vi "Old OM Setup.vi"() -> ()   [LabVIEW 2013]
uses:
  lib/Data Access Objects/Metadata/Persistant DAO Actions.ctl
  lib/Data Access Objects/Metadata/LBCB Number.ctl
  Popups/External Sensor Specs.ctl
  lib/Data Access Objects/Application/Number Of LBCBs.ctl
  Popups/Update Table Actions.ctl
  lib/Data Access Objects/Metadata/LBCB Location.ctl
  lib/Data Access Objects/Metadata/Actuator Point.ctl
  lib/Data Access Objects/Metadata/Actuator Matrix.ctl
  lib/Data Access Objects/Metadata/Cartesian Point.ctl
  lib/Data Access Objects/Metadata/Cartesian Matrix.ctl
  lib/Data Access Objects/Application/Timing Parameters.ctl
  lib/Data Access Objects/Application/App Parameters.ctl
  lib/Data Access Objects/Metadata/LBCB Position.ctl
  lib/MixedMode/Stiffness Matrix.ctl
  lib/Data Access Objects/Limits/Limit Boundary Parameters.ctl
  lib/Data Access Objects/Autobalance/Autobalance Control Parameters.ctl
  lib/Data Access Objects/Metadata/Actuator Channel Names.ctl
  lib/MixedMode/Ramp Control.ctl
  lib/MixedMode/Ramp Time Input.ctl
  lib/Data Access Objects/Metadata/Cartesian Force Vector.ctl
  lib/Data Access Objects/Application/Network Parameters.ctl
  lib/Data Access Objects/Mixed Mode/Force Control Parameters.ctl
  lib/Data Access Objects/Metadata/Cartesian Force Matrix.ctl
  lib/Data Access Objects/Metadata/Pin Positions.ctl
panel:
  out "Profile":string
  in  "Rigid Connection":bool
  in  "LBCB Number Button":bool
  in  "Number of LBCBs":T1
  in  "Save":bool
  in  "OM Setup Page Tab":T2(tab)
  in  "Act Incr Limit":T3 caption="Increment Limits"
  in  "Act Disp Bnd":T4 caption="Actuator Disp Limit \nBoundary Parameters"
  in  "Actuator Force Limits":T5
  in  "Actuator Stroke Limits":T5
  in  "Command Voltage Limit":T5
  in  "Act Force Bnd":T4 caption="Actuator Force Limit \nBoundary Parameters"
  in  "Cart Incr Limits":T6 caption="Increment Limits"
  in  "Cartesian Displacement Limits":T7
  in  "Cartesian Force Limits":T7
  in  "Cart Force Bnd":T4 caption="Cartesian Force Limit \nBoundary Parameters"
  in  "Cart Trans Bnd":T4 caption="Cartesian Translation Limit \nBoundary Parameters"
  in  "Cart Rot Bnd":T4 caption="Cartesian Rotation Limit \nBoundary Parameters"
  in  "Cart Mmt Bnd":T4 caption="Cartesian Moment Limit \nBoundary Parameters"
  in  "Auto Balance Control":T8={"Number of Samples"=0, "Delay After Cmd"=0, "Maximum Command"=0.0, "1/4 Linear Range"=0.5}
  in  "Auto Balance Error Window":T3
  in  "I Gain":T3
  in  "P Gain":T3
  in  "NTCP Network":T9={"Port Number"=0, "Notification Name"="DataAvailableForTransmission", "Wait For Notification Timeout"=1000}
  in  "DAQ Link Network":T9={"Port Number"=0, "Notification Name"="DataAvailableForTransmission", "Wait For Notification Timeout"=1000}
  in  "Application Timing and Logging":T10
  in  "Ramp Times":T12
  in  "LBCB Pin Positions":T14
  in  "LBCB Position":T15={"Motion Center"=[0.0, 0.0, 0.0], "Transformation Matrix"=[[1.0, 0.0, 0.0, 0.0, 0.0, 0.0], [0.0, 1.0, 0.0, 0.0, 0.0, 0.0], [0.0, 0.0, 1.0, 0.0, 0.0, 0.0], [0.0, 0.0, 0.0, 1.0, 0.0, 0.0], [0.0, 0.0, 0.0, 0.0, 1.0, 0.0], [0.0, 0.0, 0.0, 0.0, 0.0, 1.0]]} {"Transformation Matrix" format="%#_10e"; "Motion Center" format="%#_10g"}
  in  "Force Control Parameters":T16
  in  "Stiffness Limit":T17
  in  "Force Group Priorities":T18
  in  "Force Error Range":T18
  in  "Jacobian Gain":T6
  in  "Max Increment":T6
  in  "Stiffness Jacobian":T19=[[1000000.0, 0.0, 0.0, 0.0, 0.0, 0.0], [0.0, 1000000.0, 0.0, 0.0, 0.0, 0.0], [0.0, 0.0, 1000000.0, 0.0, 0.0, 0.0], [0.0, 0.0, 0.0, 1000000.0, 0.0, 0.0], [0.0, 0.0, 0.0, 0.0, 1000000.0, 0.0], [0.0, 0.0, 0.0, 0.0, 0.0, 1000000.0]]
  in  "Servo Error Offset":T3
  in  "LVDT  Offset":T3
  in  "Load Cell  Offset":T3
  in  "Load Cell Sensitivity":T3
  in  "Command Sensitivity":T3
  in  "LVDT Sensitivity":T3
  in  "Command Channels":T20
  in  "LVDT Channels":T20
  in  "Load Cell Channels":T20
  in  "Servo Error  Channels":T20
  in  "External Sensor Specs":T21[](array[typedef])
  out "OM  Location":T22
  in  "Ok":bool
  in  "LBCB Number":T23
  # "(Volts)"
  # "Interval is in Seconds\nRate is in Samples per Second"
  # "Fixed"
  # "Platten"
  # "X"
  # "Z"
  # "X"
  # "Z"
  # "Y"
  # "Y"
  # "Y"
  # "(inch)"
  # "XLBCB CMD = T-1*XLBCB OM"
  # "Z"
  # "(inch)"
  # "XOM DISP = T*XLBCB DISP"
  # "(inch)"
  # "Dx"
  # "Dy"
  # "Dz"
  # "Rx"
  # "Ry"
  # "Rz"
  # "Dx"
  # "Dy"
  # "Dz"
  # "Rx"
  # "Ry"
  # "Rz"
  # "DAQMx Global Channel"
  # "Display Name"
  # "Sensiitivity"
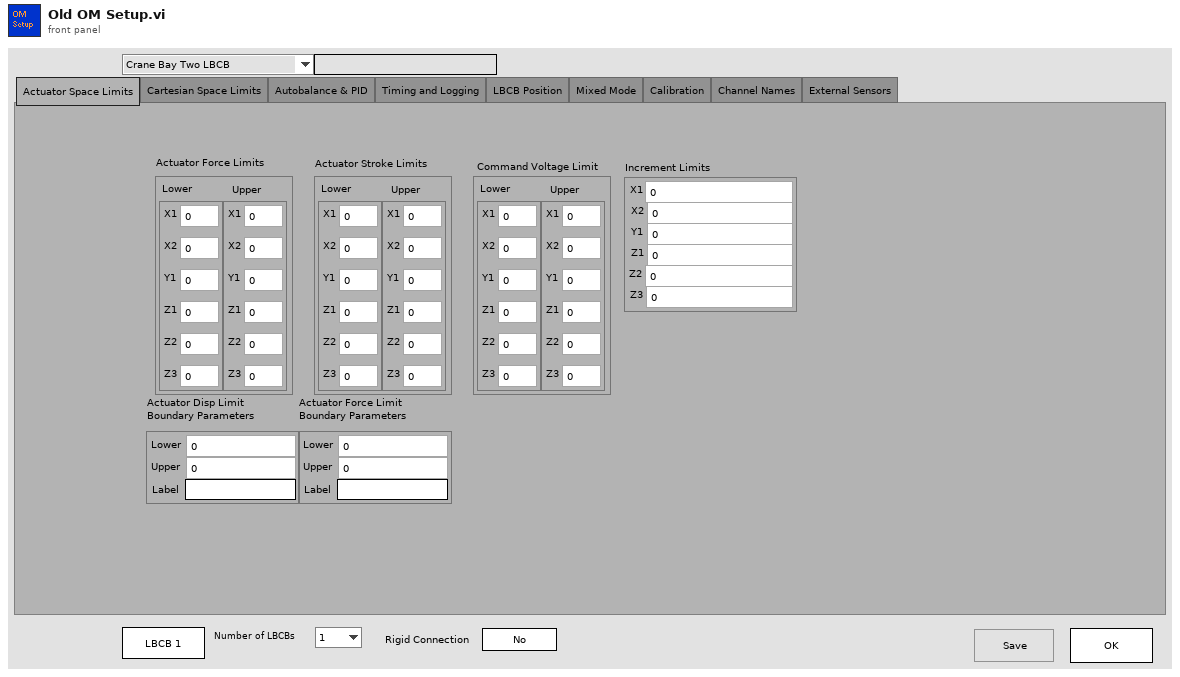
[diagram p1: front panel]
types:
  T1 = typedef "Number Of LBCBs.ctl" = enum16{"1", "2"}
  T2 = enum32{"Actuator Space Limits", "Cartesian Space Limits", "Autobalance & PID", "Timing and Logging", "LBCB Position", "Mixed Mode", "Calibration", "Channel Names", "External Sensors"}
  T3 = typedef "Actuator Point.ctl" = cluster{"X1":dbl, "X2":dbl, "Y1":dbl, "Z1":dbl, "Z2":dbl, "Z3":dbl}
  T4 = typedef "Limit Boundary Parameters.ctl" = cluster{"Lower":dbl, "Upper":dbl, "Label":string}
  T5 = typedef "Actuator Matrix.ctl" = cluster{"Lower":T3, "Upper":T3}
  T6 = typedef "Cartesian Point.ctl" = cluster{"Dx":dbl, "Dy":dbl, "Dz":dbl, "Rx":dbl, "Ry":dbl, "Rz":dbl}
  T7 = typedef "Cartesian Matrix.ctl" = cluster{"Lower":T6, "Upper":T6}
  T8 = typedef "Autobalance Control Parameters.ctl" = cluster{"Number of Samples":i32, "Delay After Cmd":i32, "Maximum Command":dbl, "1/4 Linear Range":dbl}
  T9 = typedef "Network Parameters.ctl" = cluster{"Port Number":u16, "Notification Name":string, "Wait For Notification Timeout":i32}
  T10 = typedef "App Parameters.ctl" = cluster{"Monitor Loop":T11, "Ramp Time":T11, "Log Loop":T11, "TCP to DAQ":T11, "Logging Directory":path, "Log File Size (MBytes)":i64, "Volt Logging Loop":T11, "2 LBCB Archiving Mode":bool, "Fake":bool}
  T11 = typedef "Timing Parameters.ctl" = cluster{"Interval":dbl, "Rate ":dbl}
  T12 = typedef "Ramp Time Input.ctl" = cluster{"Directional":T13, "Iterative":T13}
  T13 = typedef "Ramp Control.ctl" = cluster{"Ramp":dbl, "Stabilize":dbl, "Hold":dbl}
  T14 = typedef "Pin Positions.ctl" = cluster{"Pin Positions":dbl[][], "Row Labels":string[]}
  T15 = typedef "LBCB Position.ctl" = cluster{"Motion Center":dbl[], "Transformation Matrix":dbl[][]}
  T16 = typedef "Force Control Parameters.ctl" = cluster{"Use Force Error Range Ratios":bool, "Use Group Priorities":bool, "Multi Command Update":bool, "Steps per Stiffness \nMeasurement":i32}
  T17 = typedef "Cartesian Force Matrix.ctl" = cluster{"Lower":T18, "Upper":T18}
  T18 = typedef "Cartesian Force Vector.ctl" = cluster{"Fx":dbl, "Fy":dbl, "Fz":dbl, "Mx":dbl, "My":dbl, "Mz":dbl}
  T19 = typedef "Stiffness Matrix.ctl" = dbl[][]
  T20 = typedef "Actuator Channel Names.ctl" = cluster{"X1":refnum<k21>, "X2":refnum<k21>, "Y1":refnum<k21>, "Z1":refnum<k21>, "Z2":refnum<k21>, "Z3":refnum<k21>}
  T21 = typedef "External Sensor Specs.ctl" = cluster{"DAQmx Global Channel":refnum<k21>, "Display Name":string, "Sensitivity":dbl}
  T22 = typedef "LBCB Location.ctl" = enum16{"Crane Bay Two LBCB", "Crane Bay One LBCB", "5th Scale Two LBCB", "5th Scale One LBCB", "Portable LBCB", "University of Houston LBCB"}
  T23 = typedef "LBCB Number.ctl" = enum16{"LBCB1", "LBCB2"}
  T24 = typedef "Persistant DAO Actions.ctl" = enum16{"Init", "Get", "Set", "Load", "Save"}
  T25 = typedef "Update Table Actions.ctl" = enum16{"Update Table", "Exit"}
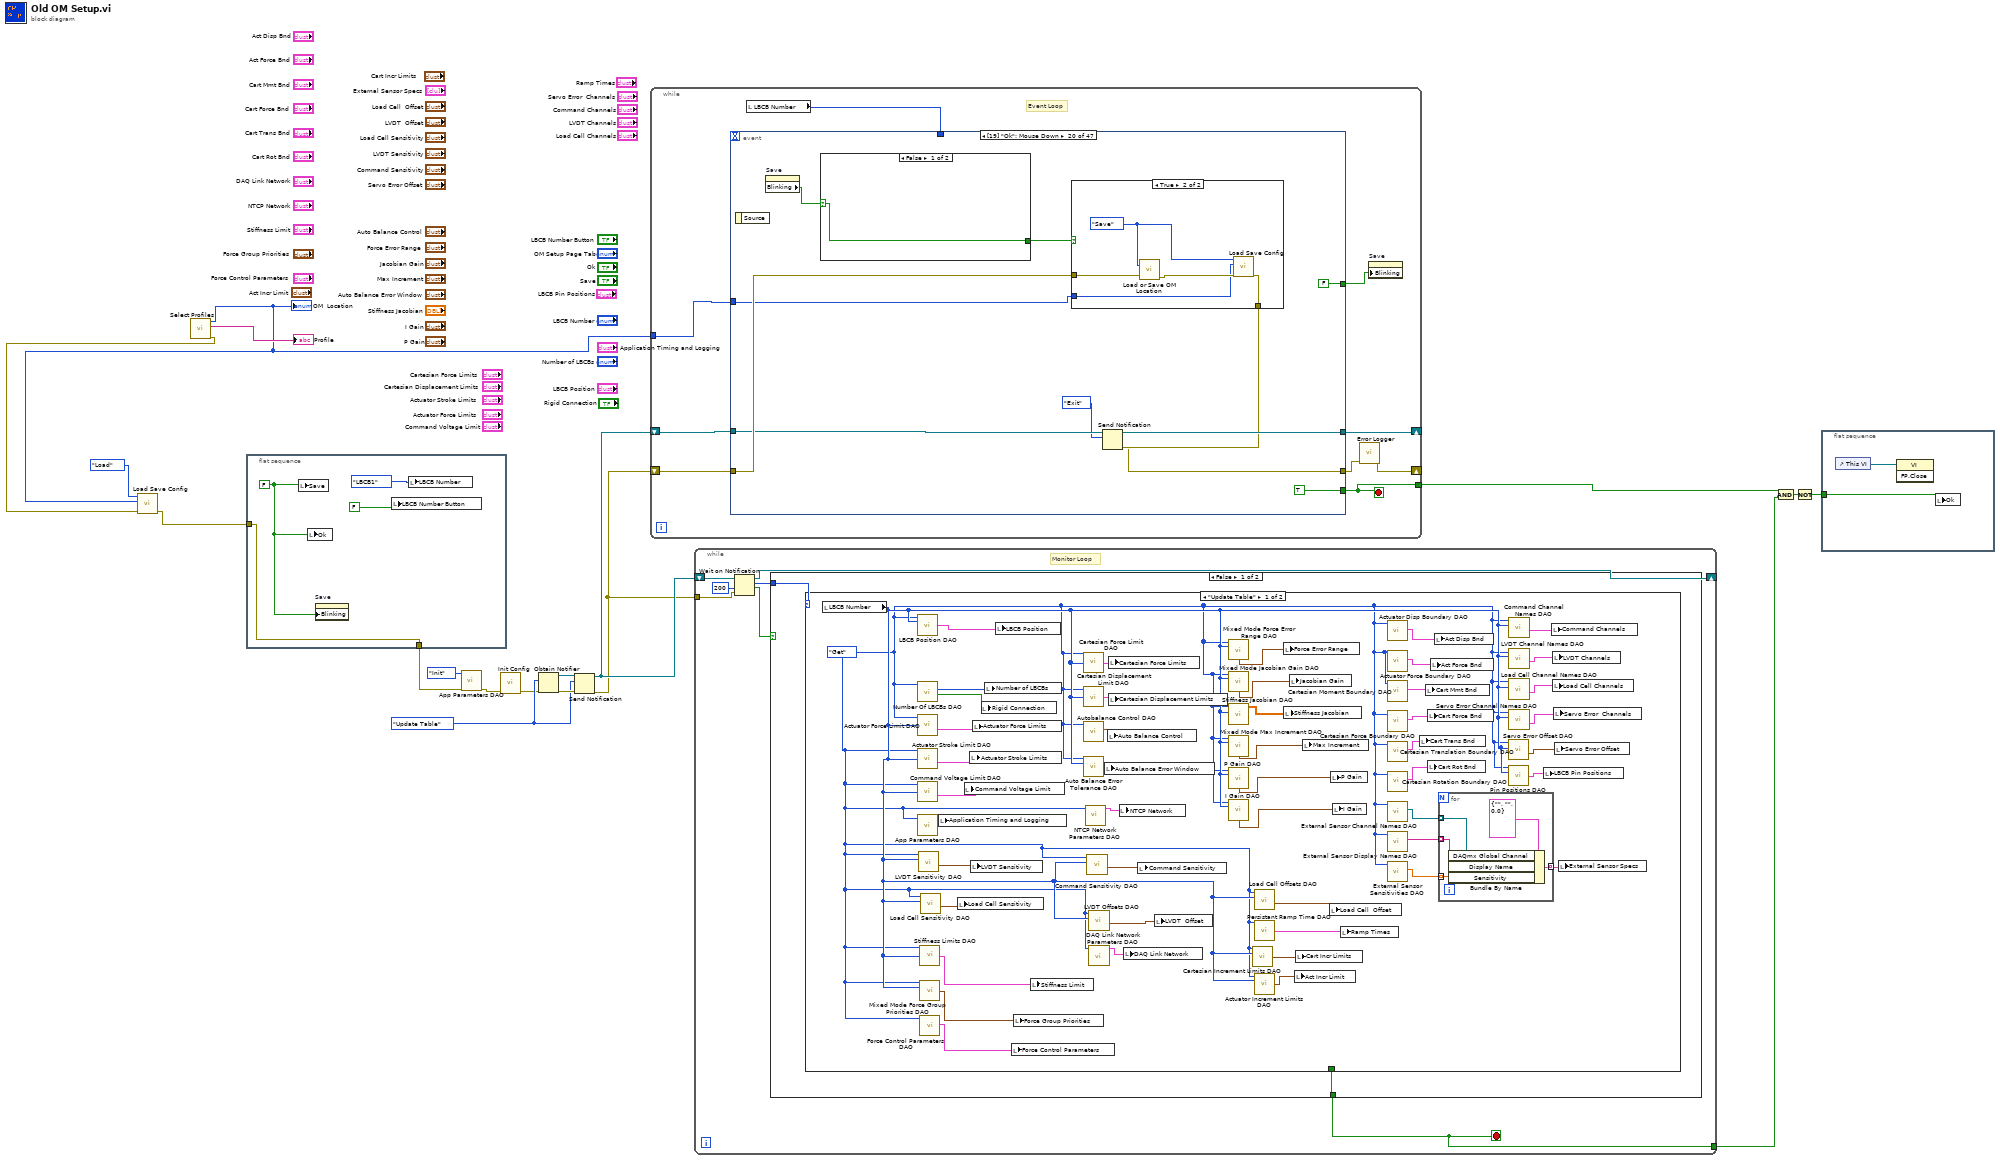
[diagram p0: block diagram]
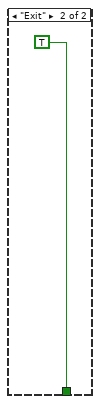
[diagram p2: hidden frame]
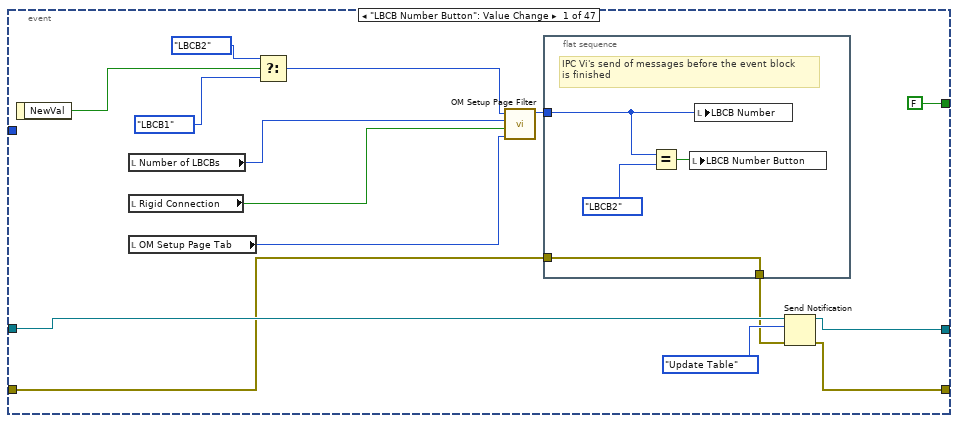
[diagram p4: hidden frame]
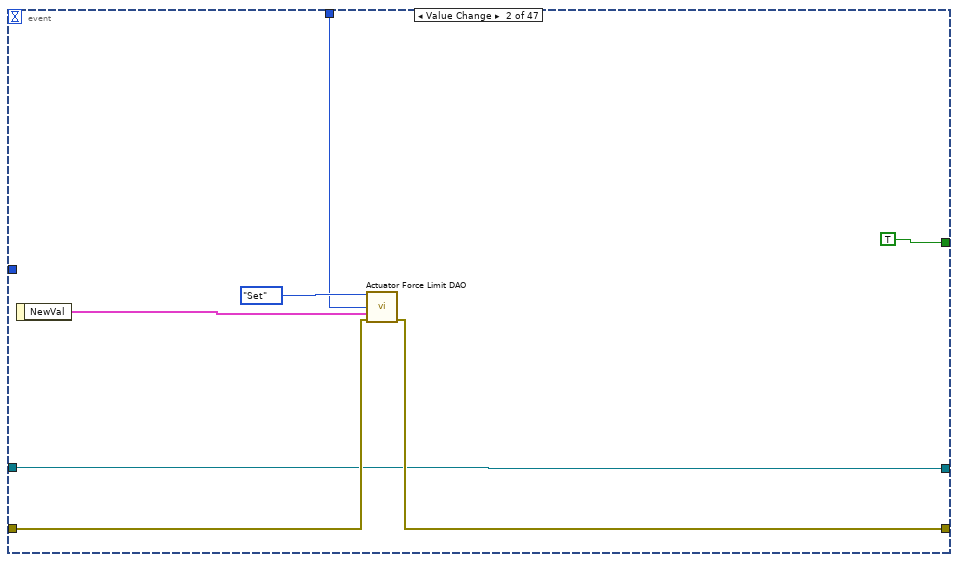
[diagram p5: hidden frame]
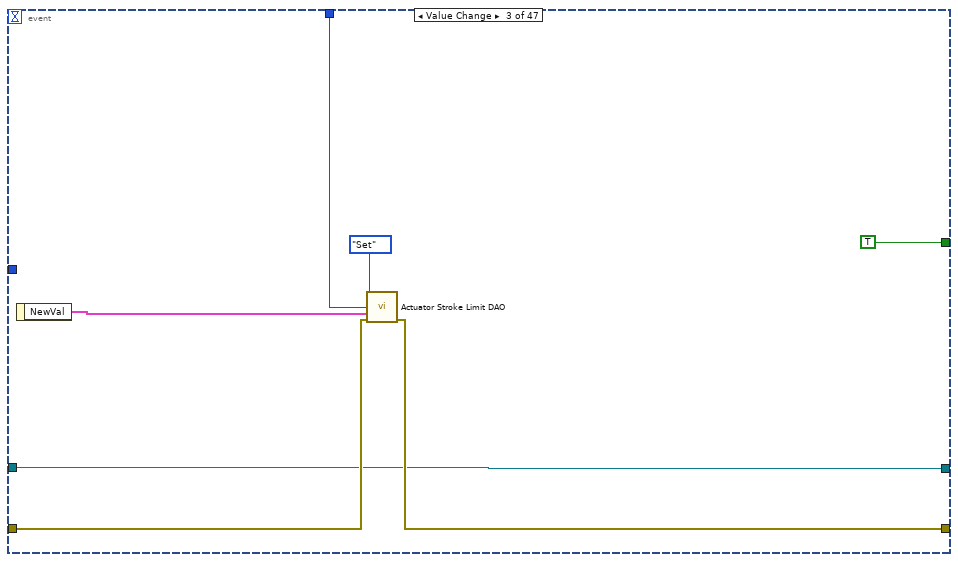
[diagram p6: hidden frame]
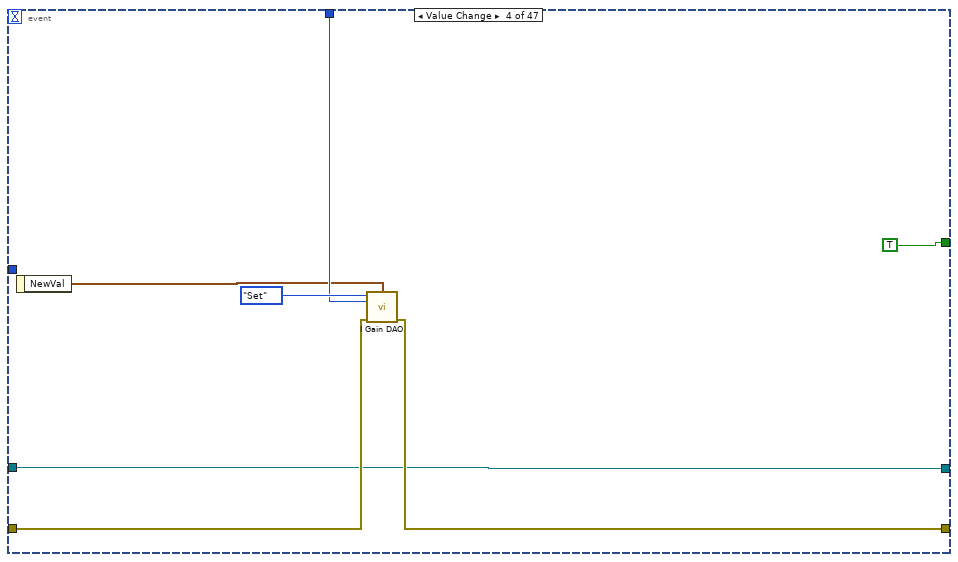
[diagram p7: hidden frame]
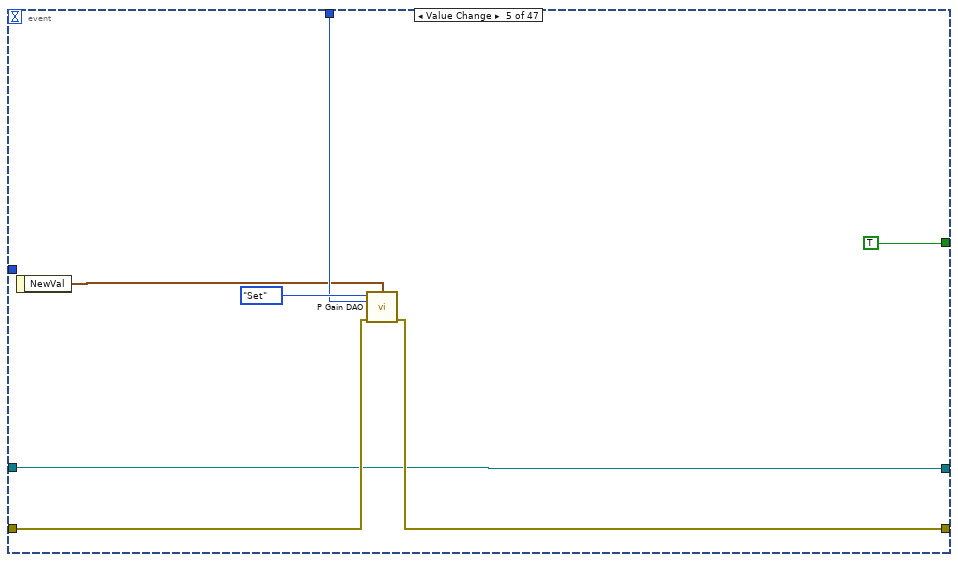
[diagram p8: hidden frame]
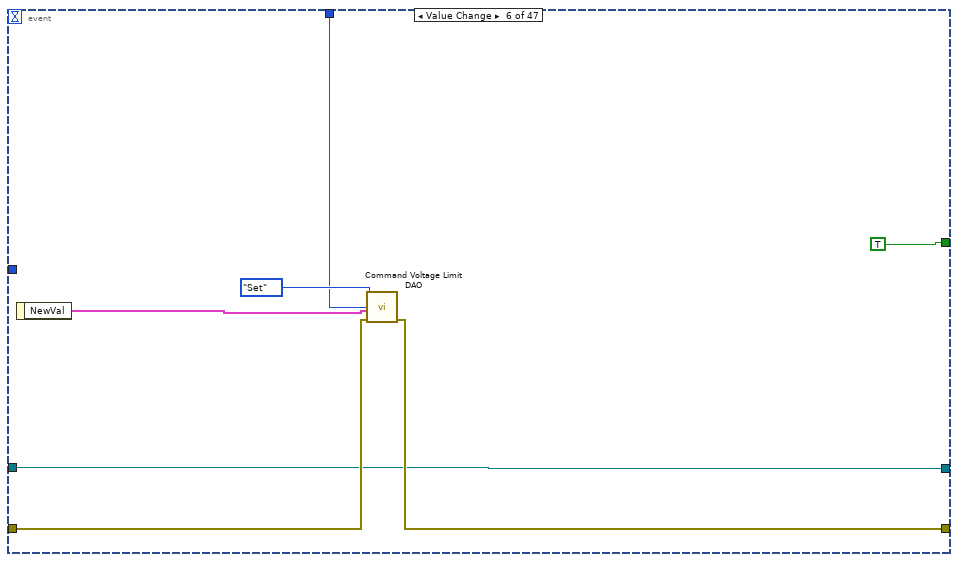
[diagram p9: hidden frame]
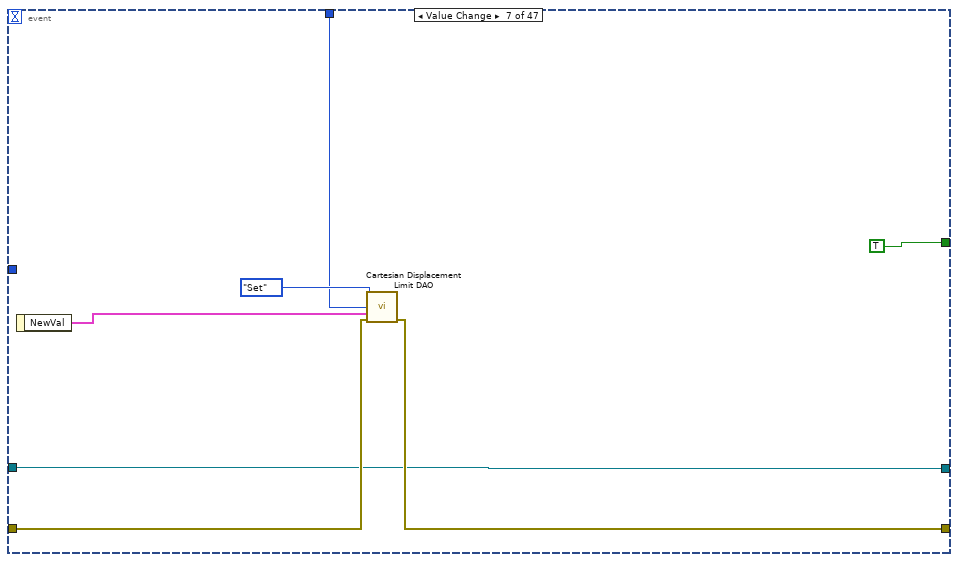
[diagram p10: hidden frame]
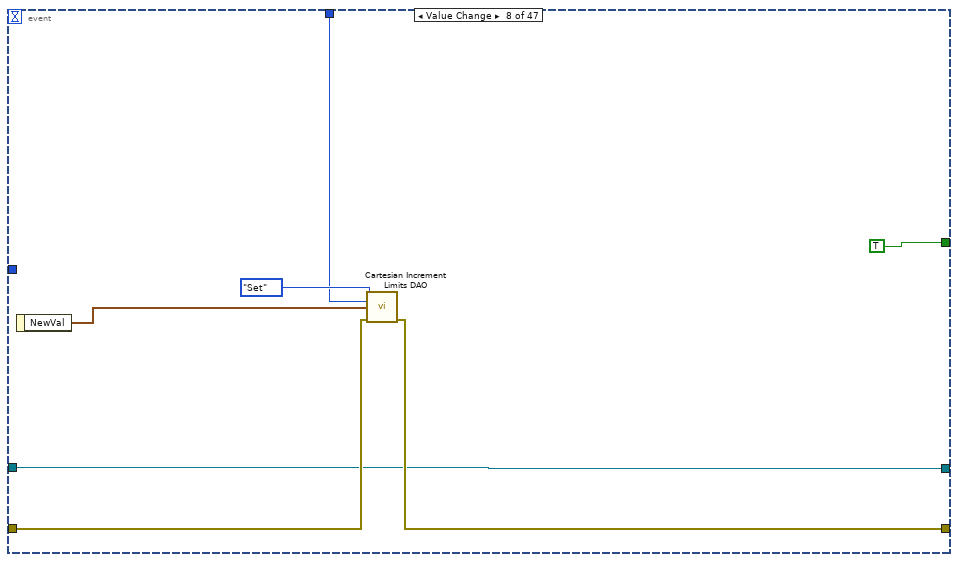
[diagram p11: hidden frame]
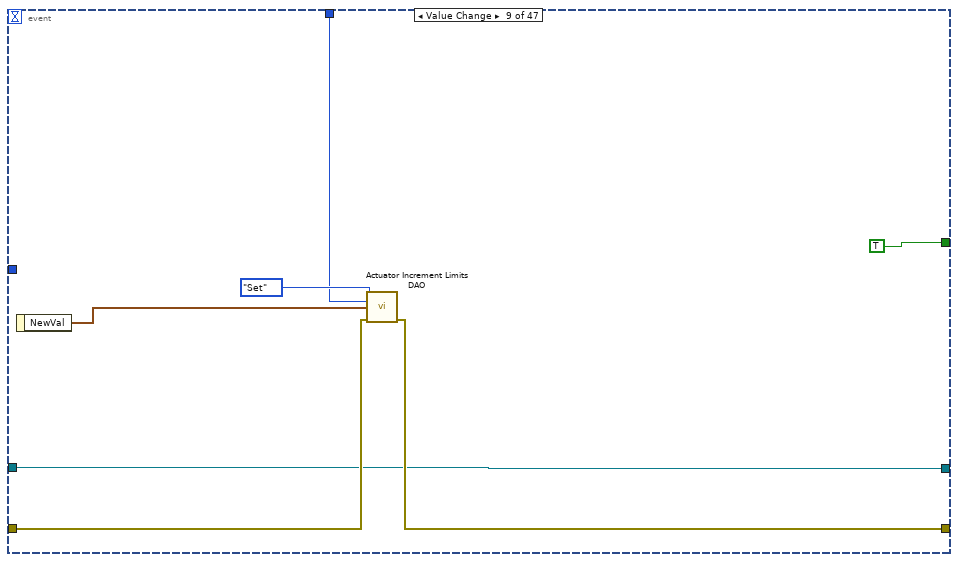
[diagram p12: hidden frame]
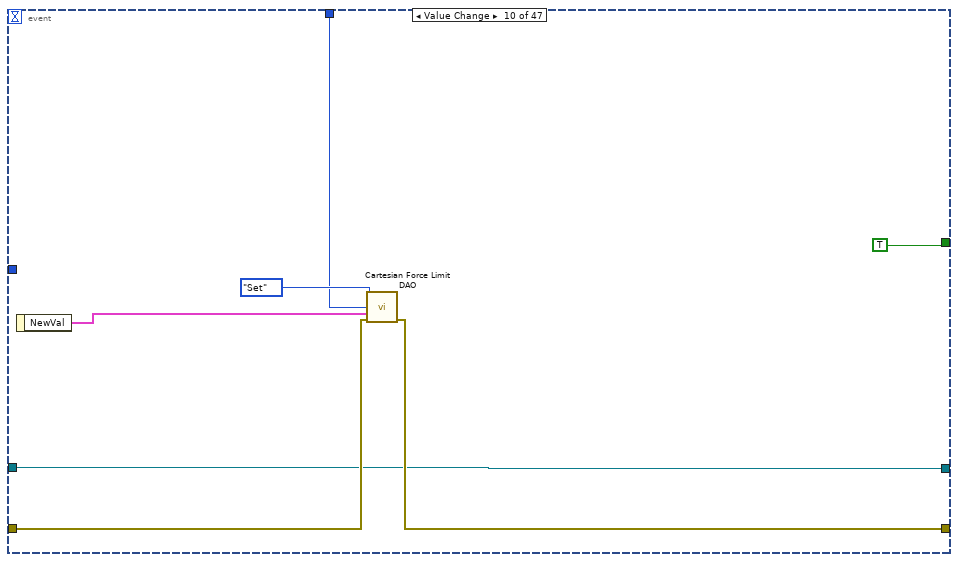
[diagram p13: hidden frame]
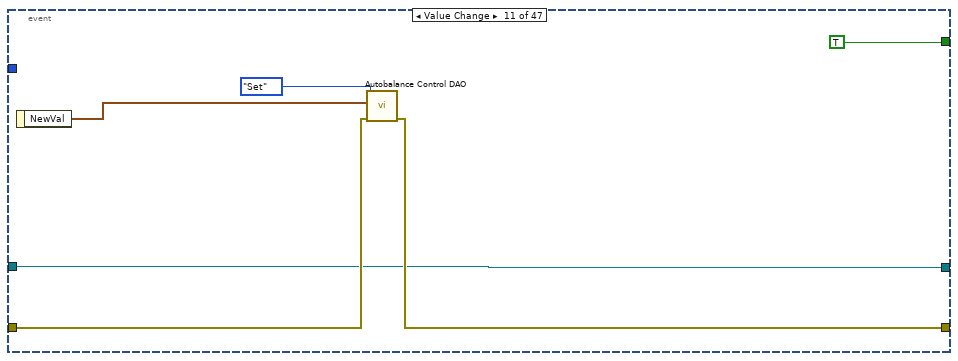
[diagram p14: hidden frame]
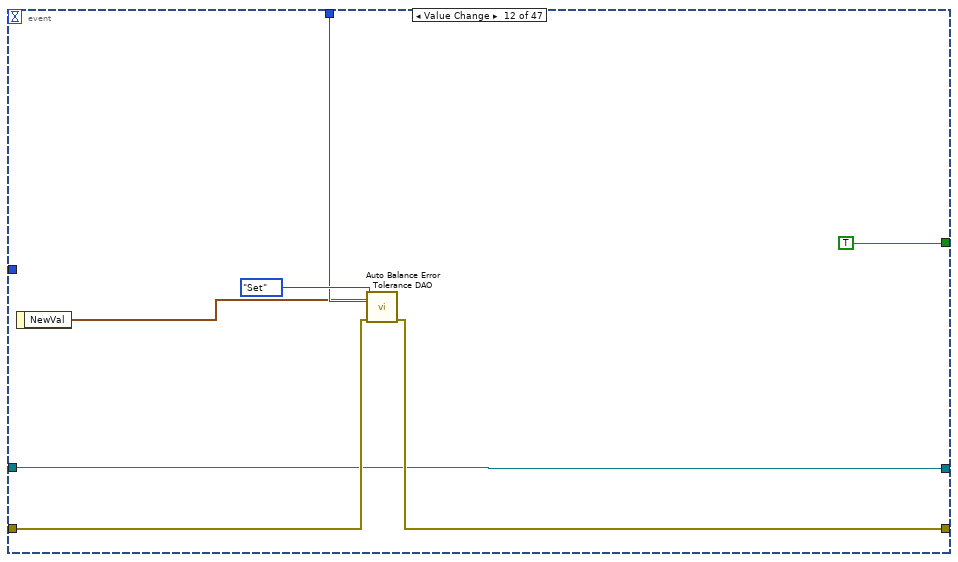
[diagram p15: hidden frame]
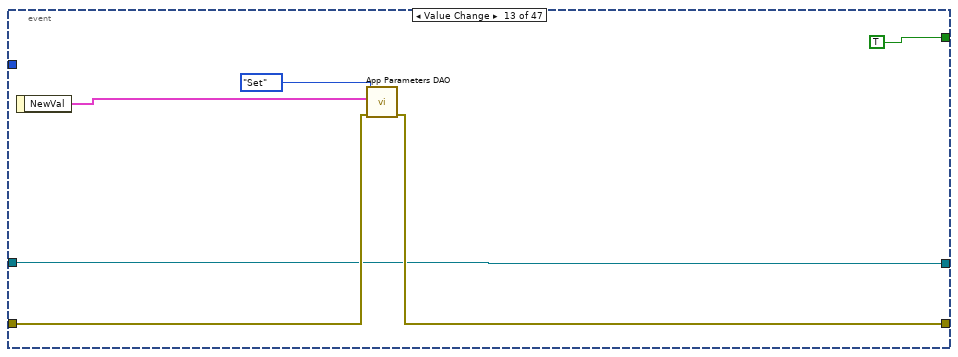
[diagram p16: hidden frame]
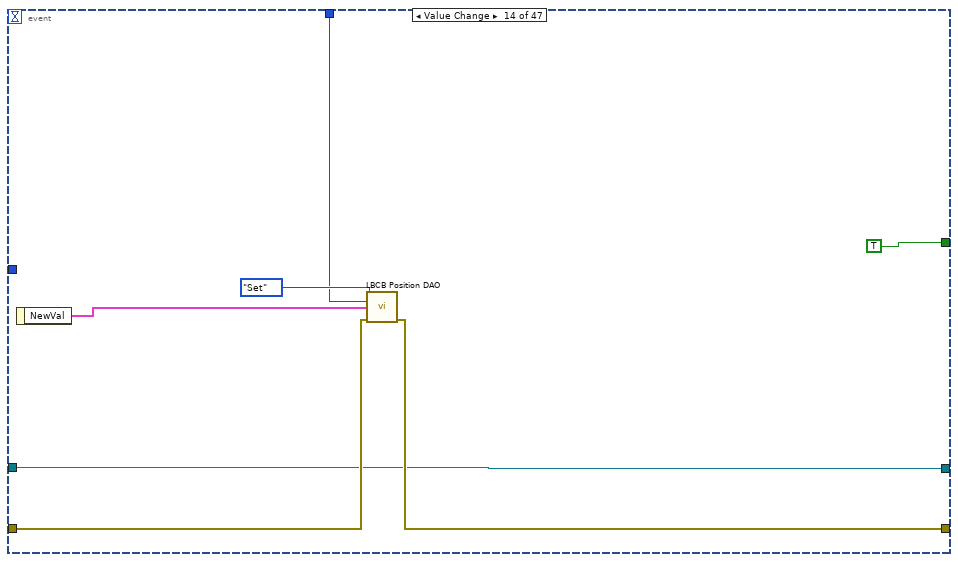
[diagram p17: hidden frame]
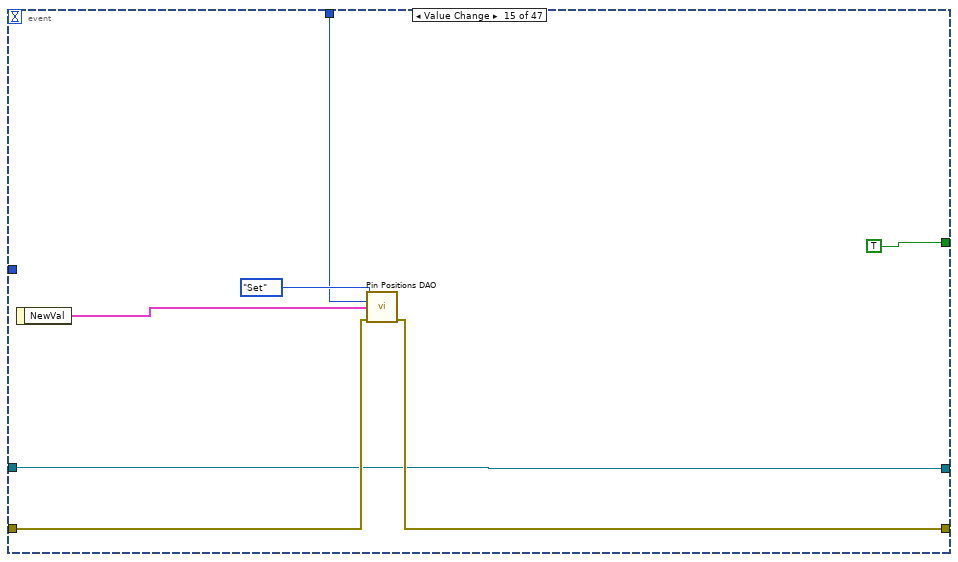
[diagram p18: hidden frame]
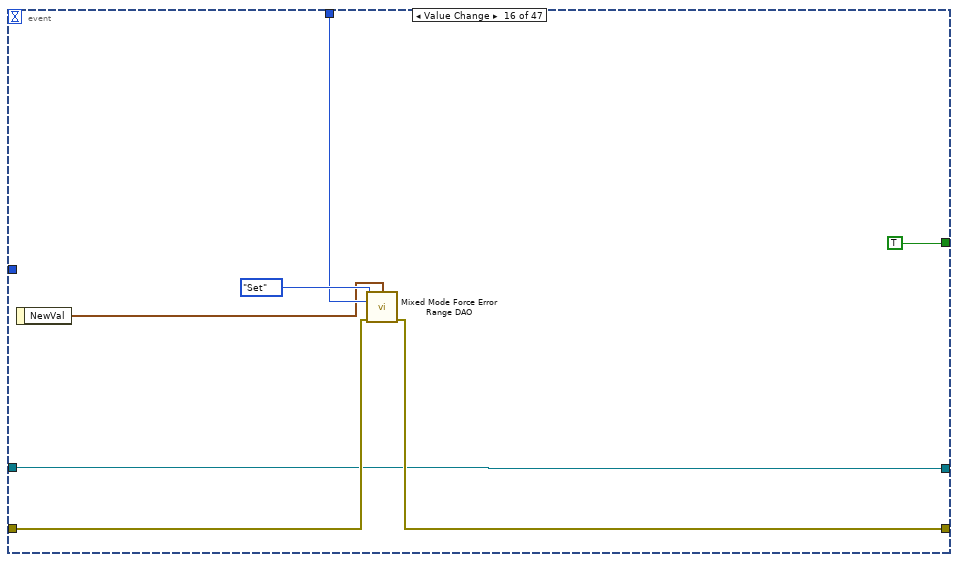
[diagram p19: hidden frame]
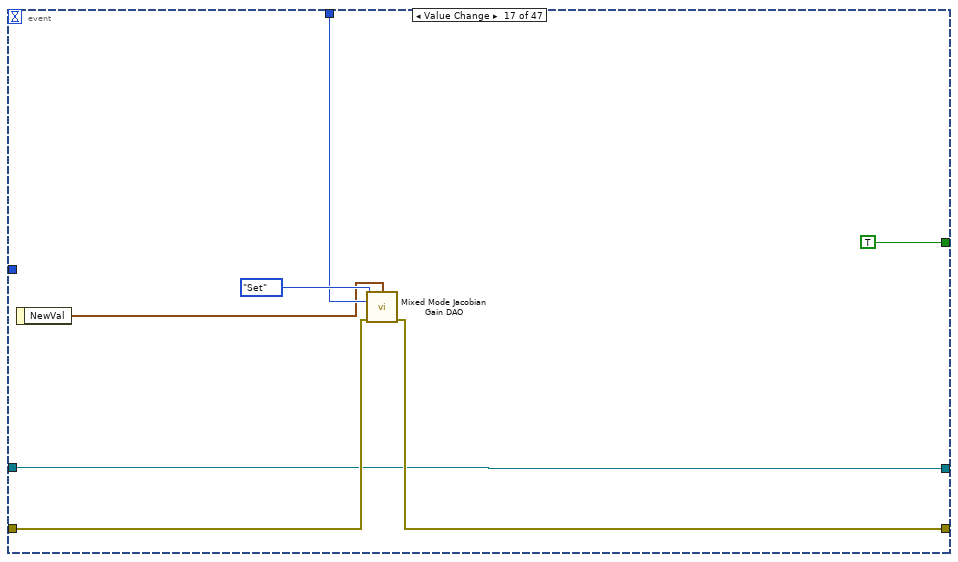
[diagram p20: hidden frame]
diagram:
  w16 = Update_Table_Actions."Update Table" ("Update Actions")
  n1 = call "Select Profiles.vi"() -> ("error out"=w2:errorcluster, "Profile Out"=→"Profile":string, "LBCB  Location Out"=w3:T22)  [unwired: 9 in]
  "OM  Location" <- w3
  n2 = call "Load Save Config.vi"("error in (no error)"=w2, "OM  Location"=w3, "Actions"=Persistant_DAO_Actions."Load") -> ("error out"=w5:errorcluster)  [unwired: 1 in, 7 out]
  n3 = flat-sequence {
    tunnel: w5 -> [w19]
    tunnel: [w19] -> w1
    frame #0 {
      w20 = FALSE ("Save")
      n4 = local write "Save"(w20) -> ()
      n5 = local write "Ok"(w20) -> ()
      n6 = property on="Save" class="Bool (strict)"("Blinking"=w20) -> ()  [unwired: 2 in, 2 out]
      n7 = local write "LBCB Number Button"(FALSE ("LBCB Number Button")) -> ()
      n8 = local write "LBCB Number"(LBCB_Number."LBCB1" ("LBCB Number")) -> ()
    }
  }
  n9 = call "App Parameters DAO.vi"("error in (no error)"=w1, "Actions"=Persistant_DAO_Actions."Init") -> ("error out"=w8:errorcluster)  [unwired: 7 in, 2 out]
  n10 = call "Init Config.vi"("error in (no error)"=w8) -> ("error out"=w13:errorcluster)  [unwired: 10 out]
  n11 = Obtain Notifier(notification data type=w16, error in (no error)=w13) -> (notifier out=w18:refnum<notifier>, error out=w17:errorcluster)  [unwired: 1 in, 2 out]
  n12 = Send Notification(notification=w16, notifier=w18, error in (no error)=w17) -> (notifier out=w15:refnum<notifier>, error out=w14:errorcluster)
  n13 = while {
    shift-right: [w29] -> _
    shift-left: w14 -> [w31]
    shift-right: [w27] -> _
    shift-left: w15 -> [w28]
    tunnel: [w24] -> w12
    tunnel: w3 -> [w23]
    stop <- w24 stop-if-true
    # "Event Loop"
    n14 = local read "LBCB Number"() -> (w26:T23)
    n15 = event shown="[19] \"Ok\": Mouse Down" {
      selector: _ -> [_ _ _ _ _ _ _ _ _ _ _ _ _ _ _ _ _ _ _ _ _ _ _ _ _ _ _ _ _ _ _ _ _ _ _ _ _ _ _ _ _ _ _ _ _ _ _]
      dyn-events: _ -> [_ _ _ _ _ _ _ _ _ _ _ _ _ _ _ _ _ _ _ _ _ _ _ _ _ _ _ _ _ _ _ _ _ _ _ _ _ _ _ _ _ _ _ _ _ _ _]
      timeout: _ -> [_ _ _ _ _ _ _ _ _ _ _ _ _ _ _ _ _ _ _ _ _ _ _ _ _ _ _ _ _ _ _ _ _ _ _ _ _ _ _ _ _ _ _ _ _ _ _]
      tunnel: w31 -> [w33 w55 w62 w69 w76 w83 w90 w97 w104 w111 w118 w124 w131 w137 w144 w151 w158 w165 w172 w188 w208 w223 w229 w235 w241 w247 w253 w260 w265 w274 w280 w287 w294 w297 w322 w329 w336 w343 w350 w356 w362 w368 w374 w381 w388 w397 w418]
      tunnel: [w46 w54 w61 w68 w75 w82 w89 w96 w103 w110 w117 w123 w130 w136 w143 w150 w157 w164 w168 w182 w207 w222 w228 w234 w240 w246 w252 w259 w264 w275 w279 w286 w293 w297 w323 w330 w337 w344 w351 w355 w361 w367 w373 w380 w387 w396 w417] -> w30
      tunnel: w28 -> [w45 w53 w60 w67 w74 w81 w88 w95 w102 w109 w116 w122 w129 w135 w142 w149 w156 w163 w175 w185 w209 w221 w227 w233 w239 w245 w251 w258 w268 w270 w277 w283 w291 w305 w318 w326 w333 w340 w347 w354 w360 w366 w372 w379 w386 w398 w416]
      tunnel: [w44 w53 w60 w67 w74 w81 w88 w95 w102 w109 w116 w122 w129 w135 w142 w149 w156 w163 w175 w184 w206 w221 w227 w233 w239 w245 w251 w258 w268 w270 w277 w283 w291 w305 w318 w326 w333 w340 w347 w354 w360 w366 w372 w379 w386 w395 w415] -> w27
      tunnel: w26 -> [_ w56 w63 w70 w77 w84 w91 w98 w105 w112 _ w125 _ w138 w145 w152 w159 w166 _ _ _ _ _ _ _ _ _ w255 w266 w272 w282 w289 w296 _ w320 w327 w334 w341 w348 _ _ _ w375 w382 _ _ w409]
      tunnel: [_ _ _ _ _ _ _ _ _ _ _ _ _ _ _ _ _ _ _ TRUE _ _ _ _ _ _ _ _ _ _ _ _ _ _ _ _ _ _ _ _ _ _ _ _ _ _ _] -> w24
      tunnel: [FALSE ("Blinking") TRUE ("Blinking") TRUE ("Blinking") TRUE ("Blinking") TRUE ("Blinking") TRUE ("Blinking") TRUE ("Blinking") TRUE ("Blinking") TRUE ("Blinking") TRUE ("Blinking") TRUE ("Blinking") TRUE ("Blinking") TRUE ("Blinking") TRUE ("Blinking") TRUE ("Blinking") TRUE ("Blinking") TRUE ("Blinking") TRUE ("Blinking") w170 FALSE ("Blinking") TRUE ("Blinking") TRUE ("Blinking") TRUE ("Blinking") TRUE ("Blinking") TRUE ("Blinking") TRUE ("Blinking") TRUE ("Blinking") TRUE ("Blinking") TRUE ("Blinking") TRUE ("Blinking") TRUE ("Blinking") TRUE ("Blinking") TRUE ("Blinking") TRUE ("Blinking") TRUE ("Blinking") TRUE ("Blinking") TRUE ("Blinking") TRUE ("Blinking") TRUE ("Blinking") TRUE ("Blinking") TRUE ("Blinking") TRUE ("Blinking") TRUE ("Blinking") TRUE ("Blinking") TRUE ("Blinking") TRUE ("Blinking") FALSE ("Blinking")] -> w25
      tunnel: w23 -> [_ _ _ _ _ _ _ _ _ _ _ _ _ _ _ _ _ _ w171 w178 _ _ _ _ _ _ _ _ _ _ _ _ _ _ _ _ _ _ _ _ _ _ _ _ _ _ _]
      event "LBCB Number Button": Value Change {
        n16 = event-data() -> ("NewVal"=w39:bool)  [unwired: 1 out]
        n17 = local read "Number of LBCBs"() -> (w37:T1)
        n18 = local read "Rigid Connection"() -> (w36:bool)
        n19 = local read "OM Setup Page Tab"() -> (w35:T2)
        n20 = Select(t=LBCB_Number."LBCB2", s=w39, f=LBCB_Number."LBCB1" ("LBCB Number")) -> (s? t:f=w38:T23)
        n21 = call "OM Setup Page Filter.vi"("OM Setup Page"=w35, "Rigid Connection In"=w36, "Number of\nLBCBs In"=w37, "LBCB Number In"=w38) -> ("LBCB Number Out"=w34:T23)  [unwired: 7 in]
        n22 = flat-sequence {
          tunnel: w34 -> [w49]
          tunnel: w33 -> [w47]
          tunnel: [w47] -> w32
          frame #0 {
            # "IPC Vi's send of messages before the event block\nis finished"
            n23 = Equal?(x=w49, y=LBCB_Number."LBCB2") -> (x = y?=w50:bool)
            n24 = local write "LBCB Number Button"(w50) -> ()
            n25 = local write "LBCB Number"(w49) -> ()
          }
        }
        n26 = Send Notification(notification=Update_Table_Actions."Update Table", notifier=w45, error in (no error)=w32) -> (notifier out=w44:refnum<notifier>, error out=w46:errorcluster)
      }
      event Value Change {
        n27 = event-data() -> ("NewVal"=w52:T5)  [unwired: 1 out]
        n28 = call "Actuator Force Limit DAO.vi"("Actuator Force Limit Actions"=Persistant_DAO_Actions."Set" ("Actions"), "ID"=w56, "Actuator Force Limits  Input"=w52, "error in (no error)"=w55) -> ("error out"=w54:errorcluster)  [unwired: 1 in, 10 out]
      }
      event Value Change {
        n29 = event-data() -> ("NewVal"=w59:T5)  [unwired: 1 out]
        n30 = call "Actuator Stroke Limit DAO.vi"("Actuator Stroke Limit Actions"=Persistant_DAO_Actions."Set" ("Actions"), "ID"=w63, "Actuator Stroke Limits In"=w59, "error in (no error)"=w62) -> ("error out"=w61:errorcluster)  [unwired: 1 in, 10 out]
      }
      event Value Change {
        n31 = event-data() -> ("NewVal"=w66:T3)  [unwired: 1 out]
        n32 = call "I Gain DAO.vi"("I Gain Actions"=Persistant_DAO_Actions."Set" ("Actions"), "I Gain In"=w66, "LBCB Number"=w70, "error in (no error)"=w69) -> ("error out"=w68:errorcluster)  [unwired: 2 in, 9 out]
      }
      event Value Change {
        n33 = event-data() -> ("NewVal"=w73:T3)  [unwired: 1 out]
        n34 = call "P Gain DAO.vi"("P Gain Actions"=Persistant_DAO_Actions."Set" ("Actions"), "P Gain In"=w73, "LBCB Number"=w77, "error in (no error)"=w76) -> ("error out"=w75:errorcluster)  [unwired: 1 in, 10 out]
      }
      event Value Change {
        n35 = event-data() -> ("NewVal"=w80:T5)  [unwired: 1 out]
        n36 = call "Command Voltage Limit DAO.vi"("Actuator Stroke Limit Actions"=Persistant_DAO_Actions."Set" ("Actions"), "ID"=w84, "Command Voltage Limit In"=w80, "error in (no error)"=w83) -> ("error out"=w82:errorcluster)  [unwired: 2 in, 9 out]
      }
      event Value Change {
        n37 = event-data() -> ("NewVal"=w87:T7)  [unwired: 1 out]
        n38 = call "Cartesian Displacement Limit DAO.vi"("Cartesian Displacement Limit Actions"=Persistant_DAO_Actions."Set" ("Actions"), "ID"=w91, "Cartesian Displacement In"=w87, "error in (no error)"=w90) -> ("error out"=w89:errorcluster)  [unwired: 1 in, 10 out]
      }
      event Value Change {
        n39 = event-data() -> ("NewVal"=w93:T6)  [unwired: 1 out]
        n40 = call "Cartesian Increment Limits DAO.vi"("Actions"=Persistant_DAO_Actions."Set", "LBCB Number"=w98, "Inc Limits In"=w93, "error in (no error)"=w97) -> ("error out"=w96:errorcluster)  [unwired: 9 in, 2 out]
      }
      event Value Change {
        n41 = event-data() -> ("NewVal"=w100:T3)  [unwired: 1 out]
        n42 = call "Actuator Increment Limits DAO.vi"("Actions"=Persistant_DAO_Actions."Set", "LBCB Number"=w105, "Inc Limits In"=w100, "error in (no error)"=w104) -> ("error out"=w103:errorcluster)  [unwired: 9 in, 2 out]
      }
      event Value Change {
        n43 = event-data() -> ("NewVal"=w108:T7)  [unwired: 1 out]
        n44 = call "Cartesian Force Limit DAO.vi"("Cartesian Force Limit Actions"=Persistant_DAO_Actions."Set" ("Actions"), "ID"=w112, "Cartesian Force Limit In"=w108, "error in (no error)"=w111) -> ("error out"=w110:errorcluster)  [unwired: 1 in, 10 out]
      }
      event Value Change {
        n45 = event-data() -> ("NewVal"=w114:T8)  [unwired: 1 out]
        n46 = call "Autobalance Control DAO.vi"("error in (no error)"=w118, "Autobalance Control In"=w114, "Persistent DAO Actions"=Persistant_DAO_Actions."Set" ("Actions")) -> ("error out"=w117:errorcluster)  [unwired: 2 in, 6 out]
      }
      event Value Change {
        n47 = event-data() -> ("NewVal"=w121:T3)  [unwired: 1 out]
        n48 = call "Auto Balance Error Tolerance DAO.vi"("Auto Balance Increment Actions"=Persistant_DAO_Actions."Set" ("Actions"), 2:w121, "LBCB Number"=w125, "error in (no error)"=w124) -> ("error out"=w123:errorcluster)  [unwired: 2 in, 9 out]
      }
      event Value Change {
        n49 = event-data() -> ("NewVal"=w128:T10)  [unwired: 1 out]
        n50 = call "App Parameters DAO.vi"("error in (no error)"=w131, "Application Timing and Logging In"=w128, "Actions"=Persistant_DAO_Actions."Set") -> ("error out"=w130:errorcluster)  [unwired: 1 in, 7 out]
      }
      event Value Change {
        n51 = event-data() -> ("NewVal"=w134:T15)  [unwired: 1 out]
        n52 = call "LBCB Position DAO.vi"("LBCB Settings Actions"=Persistant_DAO_Actions."Set" ("Actions"), "LBCB Number"=w138, "LBCB Position In"=w134, "error in (no error)"=w137) -> ("error out"=w136:errorcluster)  [unwired: 1 in, 10 out]
      }
      event Value Change {
        n53 = event-data() -> ("NewVal"=w140:T14)  [unwired: 1 out]
        n54 = call "Pin Positions DAO.vi"("LBCB Settings Actions"=Persistant_DAO_Actions."Set" ("Actions"), "LBCB Number"=w145, "LBCB Pins In"=w140, "error in (no error)"=w144) -> ("error out"=w143:errorcluster)  [unwired: 9 in, 2 out]
      }
      event Value Change {
        n55 = event-data() -> ("NewVal"=w148:T18)  [unwired: 1 out]
        n56 = call "Mixed Mode Force Error Range DAO.vi"("Force Error Range Actions"=Persistant_DAO_Actions."Set" ("Actions"), "Force Error Range In"=w148, "LBCB Number"=w152, "error in (no error)"=w151) -> ("error out"=w150:errorcluster)  [unwired: 2 in, 9 out]
      }
      event Value Change {
        n57 = event-data() -> ("NewVal"=w155:T6)  [unwired: 1 out]
        n58 = call "Mixed Mode Jacobian Gain DAO.vi"("Jacobian Gain Actions"=Persistant_DAO_Actions."Set" ("Actions"), "Jacobian Gain In"=w155, "LBCB Number"=w159, "error in (no error)"=w158) -> ("error out"=w157:errorcluster)  [unwired: 1 in, 10 out]
      }
      event Value Change {
        n59 = event-data() -> ("NewVal"=w162:T6)  [unwired: 1 out]
        n60 = call "Mixed Mode Max Increment DAO.vi"("Max Increment Actions"=Persistant_DAO_Actions."Set" ("Actions"), "Max Increment In"=w162, "LBCB Number"=w166, "error in (no error)"=w165) -> ("error out"=w164:errorcluster)  [unwired: 1 in, 10 out]
      }
      event "Save": Mouse Down {
        w173 = Persistant_DAO_Actions."Save" ("Actions")
        n61 = event-data() -> ()  [unwired: 2 out]
        n62 = call "Load or Save OM Location.vi"("Action"=w173, "error in (no error)"=w172) -> ("error out"=w174:errorcluster)  [unwired: 2 out]
        n63 = call "Load Save Config.vi"("error in (no error)"=w174, "OM  Location"=w171, "Actions"=w173) -> ("error out"=w169:errorcluster)  [unwired: 1 in, 7 out]
        n64 = flat-sequence {
          tunnel: [w177] -> w170
          tunnel: w169 -> [w176]
          tunnel: [w176] -> w168
          frame #0 {
            w177 = FALSE ("Blinking")
            n65 = local write "Save"(w177) -> ()
          }
        }
      }
      event "Ok": Mouse Down {
        n66 = event-data() -> ()  [unwired: 2 out]
        n67 = property on="Save" class="Bool (strict)"() -> ("Blinking"=w179:bool)  [unwired: 2 in, 2 out]
        n68 = case shown="False" w179 {
          selector: w179 -> [w189 _]
          tunnel: [w189 w190] -> w187
          frame False {
          }
          frame True {
            n69 = Two Button Dialog(message="Do you want to save\nbefore loading the \nnew settings", 1:"No" ("F button name (\"Cancel\")"), 2:"Yes" ("T button name (\"OK\")")) -> (T button?=w190:bool)
          }
        }
        n70 = case shown="True" w187 {
          tunnel: [w194 w199] -> w183
          tunnel: w188 -> [w194 w196]
          tunnel: w178 -> [_ w195]
          frame False {
          }
          frame True {
            w197 = Persistant_DAO_Actions."Save" ("Actions")
            n71 = call "Load or Save OM Location.vi"("Action"=w197, "error in (no error)"=w196) -> ("error out"=w198:errorcluster)  [unwired: 2 out]
            n72 = call "Load Save Config.vi"("error in (no error)"=w198, "OM  Location"=w195, "Actions"=w197) -> ("error out"=w199:errorcluster)  [unwired: 1 in, 7 out]
          }
        }
        n73 = Send Notification(notification=Update_Table_Actions."Exit", notifier=w185, error in (no error)=w183) -> (notifier out=w184:refnum<notifier>, error out=w182:errorcluster)
      }
      event Value Change {
        n74 = event-data() -> ("NewVal"=w203:T1)  [unwired: 1 out]
        n75 = local read "Rigid Connection"() -> (w202:bool)
        n76 = Select(t=Number_Of_LBCBs."2", s=w202, f=w203) -> (s? t:f=w200:T1)
        n77 = case shown="\"1\", Default" w200 {
          tunnel: w209 -> [w214 w218]
          tunnel: w208 -> [w213 w217]
          tunnel: [w212 w217] -> w207
          tunnel: [w211 w218] -> w206
          frame "1", Default {
            n78 = local write "LBCB Number Button"(FALSE ("LBCB Number Button")) -> ()
            n79 = local write "LBCB Number"(LBCB_Number."LBCB1" ("LBCB Number")) -> ()
            n80 = Send Notification(notification=Update_Table_Actions."Update Table", notifier=w214, error in (no error)=w213) -> (notifier out=w211:refnum<notifier>, error out=w212:errorcluster)
          }
          frame "2" {
          }
        }
        n81 = local write "Number of LBCBs"(w200) -> ()
        n82 = call "Number Of LBCBs DAO.vi"("Rigid Connection In"=w202, "Number of\nLBCBs In"=w200, "Actions"=Persistant_DAO_Actions."Set") -> ()  [unwired: 2 in, 7 out]
      }
      event Value Change {
        n83 = event-data() -> ("NewVal"=w219:T4)  [unwired: 1 out]
        n84 = call "Actuator Disp Boundary DAO.vi"("error in (no error)"=w223, "Limit Boundary Parameters In"=w219, "Actions"=Persistant_DAO_Actions."Set") -> ("error out"=w222:errorcluster)  [unwired: 1 in, 7 out]
      }
      event Value Change {
        n85 = event-data() -> ("NewVal"=w225:T4)  [unwired: 1 out]
        n86 = call "Actuator Force Boundary DAO.vi"("error in (no error)"=w229, "Limit Boundary Parameters In"=w225, "Actions"=Persistant_DAO_Actions."Set") -> ("error out"=w228:errorcluster)  [unwired: 1 in, 7 out]
      }
      event Value Change {
        n87 = event-data() -> ("NewVal"=w231:T4)  [unwired: 1 out]
        n88 = call "Cartesian Moment Boundary DAO.vi"("error in (no error)"=w235, "Limit Boundary Parameters In"=w231, "Actions"=Persistant_DAO_Actions."Set") -> ("error out"=w234:errorcluster)  [unwired: 1 in, 7 out]
      }
      event Value Change {
        n89 = event-data() -> ("NewVal"=w237:T4)  [unwired: 1 out]
        n90 = call "Cartesian Force Boundary DAO.vi"("error in (no error)"=w241, "Limit Boundary Parameters In"=w237, "Actions"=Persistant_DAO_Actions."Set") -> ("error out"=w240:errorcluster)  [unwired: 2 in, 6 out]
      }
      event Value Change {
        n91 = event-data() -> ("NewVal"=w243:T4)  [unwired: 1 out]
        n92 = call "Cartesian Translation Boundary DAO.vi"("error in (no error)"=w247, "Limit Boundary Parameters In"=w243, "Actions"=Persistant_DAO_Actions."Set") -> ("error out"=w246:errorcluster)  [unwired: 1 in, 7 out]
      }
      event Value Change {
        n93 = event-data() -> ("NewVal"=w249:T4)  [unwired: 1 out]
        n94 = call "Cartesian Rotation Boundary DAO.vi"("error in (no error)"=w253, "Limit Boundary Parameters In"=w249, "Actions"=Persistant_DAO_Actions."Set") -> ("error out"=w252:errorcluster)  [unwired: 1 in, 7 out]
      }
      event Value Change {
        n95 = event-data() -> ("NewVal"=w256:T19)  [unwired: 1 out]
        n96 = call "Stiffness Jacobian DAO.vi"("error in (no error)"=w260, "Stiffness Jacobian In"=w256, "LBCB Number"=w255, "Actions"=Persistant_DAO_Actions."Set") -> ("error out"=w259:errorcluster)  [unwired: 1 in, 6 out]
      }
      event Value Change {
        n97 = event-data() -> ("NewVal"=w262:T3)  [unwired: 6 out]
        n98 = call "LVDT Sensitivity DAO.vi"("error in (no error)"=w265, "LVDT Sensitivity Offset In"=w262, "LBCB Number"=w266, "Actions"=Persistant_DAO_Actions."Set") -> ("error out"=w264:errorcluster)  [unwired: 1 in, 6 out]
      }
      event Value Change {
        n99 = event-data() -> ("NewVal"=w271:T3)  [unwired: 6 out]
        n100 = call "Command Sensitivity DAO.vi"("error in (no error)"=w274, "Command Sensitivity Offset In"=w271, "LBCB Number"=w272, "Actions"=Persistant_DAO_Actions."Set") -> ("error out"=w275:errorcluster)  [unwired: 1 in, 6 out]
      }
      event Value Change {
        n101 = event-data() -> ("NewVal"=w278:T3)  [unwired: 6 out]
        n102 = call "Load Cell Sensitivity DAO.vi"("error in (no error)"=w280, "Load Cell Sensitivity Offset In"=w278, "LBCB Number"=w282, "Actions"=Persistant_DAO_Actions."Set") -> ("error out"=w279:errorcluster)  [unwired: 1 in, 6 out]
      }
      event Value Change {
        n103 = event-data() -> ("NewVal"=w285:T3)  [unwired: 6 out]
        n104 = call "Load Cell Offsets DAO.vi"("error in (no error)"=w287, "Load Cell Displacement Offset In"=w285, "LBCB Number"=w289, "Actions"=Persistant_DAO_Actions."Set") -> ("error out"=w286:errorcluster)  [unwired: 1 in, 6 out]
      }
      event Value Change {
        n105 = event-data() -> ("NewVal"=w290:T3)  [unwired: 1 out]
        n106 = call "LVDT Offsets DAO.vi"("error in (no error)"=w294, "LVDT Displacements Offset In"=w290, "LBCB Number"=w296, "Actions"=Persistant_DAO_Actions."Set") -> ("error out"=w293:errorcluster)  [unwired: 1 in, 6 out]
      }
      event "External Sensor Specs": Value Change {
        w300 = Persistant_DAO_Actions."Set" ("Persistent DAO Actions")
        n107 = event-data() -> ("NewVal"=w299:T21[])  [unwired: 1 out]
        n108 = Empty Array?(array=w299) -> (empty?=w298:bool)
        n109 = case shown="True" w298 {
          tunnel: w299 -> [w309 _]
          tunnel: [w308 refnum<k21>[] []] -> w303
          tunnel: [w307 string[] []] -> w302
          tunnel: [w306 dbl[] []] -> w301
          frame False {
            n110 = for {
              tunnel: w309 -> [w313] mode=indexing
              tunnel: [w312] -> w308 mode=indexing
              tunnel: [w311] -> w307 mode=indexing
              tunnel: [w310] -> w306 mode=indexing
              n111 = Unbundle By Name(w313) -> ("DAQmx Global Channel"=w312:refnum<k21>, "Display Name"=w311:string, "Sensitivity"=w310:dbl)
            }
          }
          frame True {
          }
        }
        n112 = call "External Sensor Channel Names DAO.vi"("DAQ Channel In"=w303, "Persistent DAO Actions"=w300) -> ()  [unwired: 2 in, 8 out]
        n113 = call "External Sensor Display Names DAO.vi"("Display Name In"=w302, "Persistent DAO Actions"=w300) -> ()  [unwired: 2 in, 8 out]
        n114 = call "External Sensor Sensitivities DAO.vi"("Sensitivities In"=w301, "Persistent DAO Actions"=w300) -> ()  [unwired: 2 in, 8 out]
      }
      event Value Change {
        n115 = event-data() -> ("NewVal"=w319:T20)  [unwired: 1 out]
        n116 = call "Command Channel Names DAO.vi"("error in (no error)"=w322, "Names In"=w319, "LBCB Number"=w320, "Actions"=Persistant_DAO_Actions."Set") -> ("error out"=w323:errorcluster)  [unwired: 1 in, 6 out]
      }
      event Value Change {
        n117 = event-data() -> ("NewVal"=w324:T20)  [unwired: 1 out]
        n118 = call "LVDT Channel Names DAO.vi"("error in (no error)"=w329, "Names In"=w324, "LBCB Number"=w327, "Actions"=Persistant_DAO_Actions."Set") -> ("error out"=w330:errorcluster)  [unwired: 1 in, 6 out]
      }
      event Value Change {
        n119 = event-data() -> ("NewVal"=w331:T20)  [unwired: 1 out]
        n120 = call "Load Cell Channel Names DAO.vi"("error in (no error)"=w336, "Names In"=w331, "LBCB Number"=w334, "Actions"=Persistant_DAO_Actions."Set") -> ("error out"=w337:errorcluster)  [unwired: 1 in, 6 out]
      }
      event Value Change {
        n121 = event-data() -> ("NewVal"=w338:T20)  [unwired: 1 out]
        n122 = call "Servo Error Channel Names DAO.vi"("error in (no error)"=w343, "Names In"=w338, "LBCB Number"=w341, "Actions"=Persistant_DAO_Actions."Set") -> ("error out"=w344:errorcluster)  [unwired: 1 in, 6 out]
      }
      event Value Change {
        n123 = event-data() -> ("NewVal"=w345:T3)  [unwired: 1 out]
        n124 = call "Servo Error Offset DAO.vi"("error in (no error)"=w350, "Servo Error Offset In"=w345, "LBCB Number"=w348, "Actions"=Persistant_DAO_Actions."Set") -> ("error out"=w351:errorcluster)  [unwired: 1 in, 6 out]
      }
      event Value Change {
        n125 = event-data() -> ("NewVal"=w352:T12)  [unwired: 1 out]
        n126 = call "Persistant Ramp Time DAO.vi"("Ramp Time Actions"=Persistant_DAO_Actions."Set" ("Actions"), "Ramp Time In"=w352, "error in (no error)"=w356) -> ("error out"=w355:errorcluster)  [unwired: 2 in, 10 out]
      }
      event Value Change {
        n127 = event-data() -> ("NewVal"=w358:T9)  [unwired: 1 out]
        n128 = call "DAQ Link Network Parameters DAO.vi"("error in (no error)"=w362, "Network Parameters In"=w358, "Persistent DAO Actions"=Persistant_DAO_Actions."Set" ("Actions")) -> ("error out"=w361:errorcluster)  [unwired: 6 in, 2 out]
      }
      event Value Change {
        n129 = event-data() -> ("NewVal"=w364:T9)  [unwired: 1 out]
        n130 = call "NTCP Network Parameters DAO.vi"("error in (no error)"=w368, "Network Parameters In"=w364, "Persistent DAO Actions"=Persistant_DAO_Actions."Set" ("Actions")) -> ("error out"=w367:errorcluster)  [unwired: 6 in, 2 out]
      }
      event Value Change {
        n131 = event-data() -> ("NewVal"=w370:T18)  [unwired: 1 out]
        n132 = call "Mixed Mode Force Group Priorities DAO.vi"("Force Error Range Actions"=Persistant_DAO_Actions."Set" ("Actions"), "LBCB Number"=w375, "Force Group Priorities In"=w370, "error in (no error)"=w374) -> ("error out"=w373:errorcluster)  [unwired: 9 in, 2 out]
      }
      event Value Change {
        n133 = event-data() -> ("NewVal"=w377:T17)  [unwired: 1 out]
        n134 = call "Stiffness Limits DAO.vi"("Actions"=Persistant_DAO_Actions."Set", "ID"=w382, "Stiffness Limit In"=w377, "error in (no error)"=w381) -> ("error out"=w380:errorcluster)  [unwired: 9 in, 2 out]
      }
      event Value Change {
        n135 = event-data() -> ("NewVal"=w384:T16)  [unwired: 1 out]
        n136 = call "Force Control Parameters DAO.vi"("error in (no error)"=w388, "Force Control Parameters In"=w384, "DAO Actions"=Persistant_DAO_Actions."Set" ("Actions")) -> ("error out"=w387:errorcluster)  [unwired: 6 in, 2 out]
      }
      event "Rigid Connection": Value Change {
        n137 = event-data() -> ("NewVal"=w392:bool)  [unwired: 1 out]
        n138 = local read "Number of LBCBs"() -> (w390:T1)
        n139 = case shown="True" w392 {
          tunnel: w398 -> [w401 w407]
          tunnel: w397 -> [w400 w406]
          tunnel: [w400 w405] -> w396
          tunnel: [w401 w404] -> w395
          tunnel: [w399 Number_Of_LBCBs."2" ("Number of LBCBs")] -> w391
          tunnel: w390 -> [w399 _]
          frame False {
          }
          frame True {
            n140 = Send Notification(notification=Update_Table_Actions."Update Table", notifier=w407, error in (no error)=w406) -> (notifier out=w404:refnum<notifier>, error out=w405:errorcluster)
          }
        }
        n141 = local write "Number of LBCBs"(w391) -> ()
        n142 = call "Number Of LBCBs DAO.vi"("Rigid Connection In"=w392, "Number of\nLBCBs In"=w391, "Actions"=Persistant_DAO_Actions."Set") -> ()  [unwired: 2 in, 7 out]
      }
      event "OM Setup Page Tab": Value Change {
        n143 = event-data() -> ("NewVal"=w408:T2)  [unwired: 1 out]
        n144 = local read "Number of LBCBs"() -> (w411:T1)
        n145 = local read "Rigid Connection"() -> (w410:bool)
        n146 = call "OM Setup Page Filter.vi"("OM Setup Page"=w408, "Rigid Connection In"=w410, "Number of\nLBCBs In"=w411, "LBCB Number In"=w409) -> ("LBCB Number Out"=w412:T23)  [unwired: 7 in]
        n147 = local write "LBCB Number"(w412) -> ()
        n148 = Send Notification(notification=Update_Table_Actions."Update Table", notifier=w416, error in (no error)=w418) -> (notifier out=w415:refnum<notifier>, error out=w417:errorcluster)
      }
    }
    n149 = call "Error Logger.vi"("error in (no error)"=w30) -> ("error out"=w29:errorcluster)  [unwired: 1 in, 9 out]
    n150 = property on="Save" class="Bool (strict)"("Blinking"=w25) -> ()  [unwired: 2 in, 2 out]
  }
  n151 = while {
    shift-right: [w422] -> _
    shift-left: w15 -> [w425]
    tunnel: w14 -> [w420]
    tunnel: [w419] -> w11
    stop <- w419 stop-if-true
    # "Monitor Loop"
    n152 = Wait on Notification(notifier=w425, timeout in ms (-1)=200, error in (no error)=w420) -> (notifier out=w422:refnum<notifier>, notification=w421:T25, timed out?=w423:bool)  [unwired: 2 out]
    n153 = case shown="False" w423 {
      tunnel: w421 -> [w427 _]
      tunnel: [w426 _] -> w419
      frame False {
        n154 = case shown="\"Update Table\"" w427 {
          tunnel: [_ TRUE] -> w426
          frame "Update Table" {
            w429 = Persistant_DAO_Actions."Get" ("Actions")
            n155 = local read "LBCB Number"() -> (w430:T23)
            n156 = call "LBCB Position DAO.vi"("LBCB Settings Actions"=w429, "LBCB Number"=w430) -> ("LBCB Position Output"=w475:T15)  [unwired: 3 in, 10 out]
            n157 = call "Number Of LBCBs DAO.vi"("Actions"=w429) -> ("Rigid Connection Out"=w434:bool, "Number of\nLBCBs Out"=w474:T1)  [unwired: 4 in, 5 out]
            n158 = call "Actuator Force Limit DAO.vi"("Actuator Force Limit Actions"=w429, "ID"=w430) -> ("Actuator Force Limits Out"=w470:T5)  [unwired: 3 in, 10 out]
            n159 = call "Actuator Stroke Limit DAO.vi"("Actuator Stroke Limit Actions"=w429, "ID"=w430) -> ("Actuator Stroke Limits Out"=w471:T5)  [unwired: 3 in, 10 out]
            n160 = call "Command Voltage Limit DAO.vi"("Actuator Stroke Limit Actions"=w429, "ID"=w430) -> ("Command Voltage Limit Out"=w469:T5)  [unwired: 3 in, 10 out]
            n161 = call "App Parameters DAO.vi"("Actions"=w429) -> ("Application Timing and Logging Out"=w468:T10)  [unwired: 3 in, 7 out]
            n162 = call "LVDT Sensitivity DAO.vi"("LBCB Number"=w430, "Actions"=w429) -> ("LVDT Sensitivity Offsets Out"=w454:T3)  [unwired: 3 in, 6 out]
            n163 = call "Stiffness Limits DAO.vi"("Actions"=w429, "ID"=w430) -> ("Stiffness Limit Out"=w436:T7)  [unwired: 11 in, 2 out]
            n164 = call "Mixed Mode Force Group Priorities DAO.vi"("Force Error Range Actions"=w429, "LBCB Number"=w430) -> ("Force Group Priorities Out"=w432:T18)  [unwired: 11 in, 2 out]
            n165 = call "Force Control Parameters DAO.vi"("DAO Actions"=w429) -> ("Force Control Parameters Out"=w435:T16)  [unwired: 8 in, 2 out]
            n166 = call "Load Cell Sensitivity DAO.vi"("LBCB Number"=w430, "Actions"=w429) -> ("Load Cell Sensitivity Offsets Out"=w453:T3)  [unwired: 3 in, 6 out]
            n167 = local write "Application Timing and Logging"(w468) -> ()
            n168 = local write "Load Cell Sensitivity"(w453) -> ()
            n169 = local write "Command Voltage Limit"(w469) -> ()
            n170 = local write "Actuator Stroke Limits"(w471) -> ()
            n171 = local write "LVDT Sensitivity"(w454) -> ()
            n172 = local write "Actuator Force Limits"(w470) -> ()
            n173 = local write "Rigid Connection"(w434) -> ()
            n174 = local write "Number of LBCBs"(w474) -> ()
            n175 = local write "LBCB Position"(w475) -> ()
            n176 = local write "Force Control Parameters"(w435) -> ()
            n177 = local write "Force Group Priorities"(w432) -> ()
            n178 = local write "Stiffness Limit"(w436) -> ()
            n179 = call "Cartesian Force Limit DAO.vi"("Cartesian Force Limit Actions"=w429, "ID"=w430) -> ("Cartesian Force Limit Out"=w472:T7)  [unwired: 3 in, 10 out]
            n180 = call "Cartesian Displacement Limit DAO.vi"("Cartesian Displacement Limit Actions"=w429, "ID"=w430) -> ("Cartesian Displacement Out"=w473:T7)  [unwired: 3 in, 10 out]
            n181 = call "Autobalance Control DAO.vi"("Persistent DAO Actions"=w429) -> ("Autobalance Control Out"=w445:T8)  [unwired: 3 in, 7 out]
            n182 = call "Auto Balance Error Tolerance DAO.vi"("Auto Balance Increment Actions"=w429, "LBCB Number"=w430) -> (13:w467)  [unwired: 3 in, 10 out]
            n183 = call "NTCP Network Parameters DAO.vi"("Persistent DAO Actions"=w429) -> ("Network Parameters Out"=w437:T9)  [unwired: 8 in, 2 out]
            n184 = call "Command Sensitivity DAO.vi"("LBCB Number"=w430, "Actions"=w429) -> ("Command Sensitivity Offsets Out"=w450:T3)  [unwired: 3 in, 6 out]
            n185 = call "LVDT Offsets DAO.vi"("LBCB Number"=w430, "Actions"=w429) -> ("LVDT Displacements Offsets Out"=w452:T3)  [unwired: 3 in, 6 out]
            n186 = call "DAQ Link Network Parameters DAO.vi"("Persistent DAO Actions"=w429) -> ("Network Parameters Out"=w438:T9)  [unwired: 8 in, 2 out]
            n187 = local write "Auto Balance Error Window"(w467) -> ()
            n188 = local write "Auto Balance Control"(w445) -> ()
            n189 = local write "Cartesian Force Limits"(w472) -> ()
            n190 = local write "Cartesian Displacement Limits"(w473) -> ()
            n191 = local write "NTCP Network"(w437) -> ()
            n192 = local write "DAQ Link Network"(w438) -> ()
            n193 = local write "Command Sensitivity"(w450) -> ()
            n194 = local write "LVDT  Offset"(w452) -> ()
            n195 = call "Mixed Mode Force Error Range DAO.vi"("Force Error Range Actions"=w429, "LBCB Number"=w430) -> ("Force Error Range Out"=w466:T6)  [unwired: 3 in, 10 out]
            n196 = call "Mixed Mode Jacobian Gain DAO.vi"("Jacobian Gain Actions"=w429, "LBCB Number"=w430) -> ("Jacobian Gain Out"=w465:T6)  [unwired: 3 in, 10 out]
            n197 = call "Stiffness Jacobian DAO.vi"("LBCB Number"=w430, "Actions"=w429) -> ("Stiffness Jacobian Out"=w464:T19)  [unwired: 3 in, 6 out]
            n198 = call "Mixed Mode Max Increment DAO.vi"("Max Increment Actions"=w429, "LBCB Number"=w430) -> ("Max Increment Out"=w463:T6)  [unwired: 3 in, 10 out]
            n199 = call "P Gain DAO.vi"("P Gain Actions"=w429, "LBCB Number"=w430) -> ("P Gain"=w462:T3)  [unwired: 3 in, 10 out]
            n200 = call "I Gain DAO.vi"("I Gain Actions"=w429, "LBCB Number"=w430) -> ("I Gain"=w461:T3)  [unwired: 3 in, 10 out]
            n201 = call "Cartesian Increment Limits DAO.vi"("Actions"=w429, "LBCB Number"=w430) -> ("Inc Limits Out"=w433:T6)  [unwired: 11 in, 2 out]
            n202 = call "Load Cell Offsets DAO.vi"("LBCB Number"=w430, "Actions"=w429) -> ("Load Cell Displacement Offsets Out"=w451:T3)  [unwired: 3 in, 6 out]
            n203 = call "Persistant Ramp Time DAO.vi"("Ramp Time Actions"=w429) -> ("Ramp Time Out"=w439:T12)  [unwired: 3 in, 11 out]
            n204 = call "Actuator Increment Limits DAO.vi"("Actions"=w429, "LBCB Number"=w430) -> ("Inc Limits Out"=w431:T3)  [unwired: 11 in, 2 out]
            n205 = local write "Force Error Range"(w466) -> ()
            n206 = local write "Stiffness Jacobian"(w464) -> ()
            n207 = local write "Jacobian Gain"(w465) -> ()
            n208 = local write "Act Incr Limit"(w431) -> ()
            n209 = local write "Cart Incr Limits"(w433) -> ()
            n210 = local write "Max Increment"(w463) -> ()
            n211 = local write "Load Cell  Offset"(w451) -> ()
            n212 = local write "P Gain"(w462) -> ()
            n213 = local write "I Gain"(w461) -> ()
            n214 = local write "Ramp Times"(w439) -> ()
            n215 = call "Actuator Disp Boundary DAO.vi"("Actions"=w429) -> ("Limit Boundary Parameters Out"=w460:T4)  [unwired: 3 in, 7 out]
            n216 = call "Actuator Force Boundary DAO.vi"("Actions"=w429) -> ("Limit Boundary Parameters Out"=w459:T4)  [unwired: 3 in, 7 out]
            n217 = call "Cartesian Moment Boundary DAO.vi"("Actions"=w429) -> ("Limit Boundary Parameters Out"=w458:T4)  [unwired: 3 in, 7 out]
            n218 = call "Cartesian Force Boundary DAO.vi"("Actions"=w429) -> ("Limit Boundary Parameters Out"=w457:T4)  [unwired: 3 in, 7 out]
            n219 = call "Cartesian Translation Boundary DAO.vi"("Actions"=w429) -> ("Limit Boundary Parameters Out"=w456:T4)  [unwired: 3 in, 7 out]
            n220 = call "Cartesian Rotation Boundary DAO.vi"("Actions"=w429) -> ("Limit Boundary Parameters Out"=w455:T4)  [unwired: 3 in, 7 out]
            n221 = call "External Sensor Channel Names DAO.vi"("Persistent DAO Actions"=w429) -> ("DAQ Channel Out"=w449:refnum<k21>[])  [unwired: 3 in, 7 out]
            n222 = call "External Sensor Display Names DAO.vi"("Persistent DAO Actions"=w429) -> ("Display Name Out"=w448:string[])  [unwired: 3 in, 7 out]
            n223 = call "External Sensor Sensitivities DAO.vi"("Persistent DAO Actions"=w429) -> ("Sensitivities Out"=w447:dbl[])  [unwired: 3 in, 7 out]
            n224 = local write "Cart Trans Bnd"(w456) -> ()
            n225 = local write "Cart Mmt Bnd"(w458) -> ()
            n226 = local write "Cart Rot Bnd"(w455) -> ()
            n227 = local write "Cart Force Bnd"(w457) -> ()
            n228 = local write "Act Force Bnd"(w459) -> ()
            n229 = local write "Act Disp Bnd"(w460) -> ()
            n230 = for {
              tunnel: w449 -> [w479] mode=indexing
              tunnel: w448 -> [w478] mode=indexing
              tunnel: w447 -> [w477] mode=indexing
              tunnel: [w476] -> w446 mode=indexing
              n231 = Bundle By Name(cluster=T21 {"DAQmx Global Channel"="", "Display Name"="", "Sensitivity"=0.0} ("External Sensor Spec"), "DAQmx Global Channel"=w479, "Display Name"=w478, "Sensitivity"=w477) -> (w476:T21)
            }
            n232 = call "Servo Error Offset DAO.vi"("LBCB Number"=w430, "Actions"=w429) -> ("Servo Error  Offsets Out"=w440:T3)  [unwired: 3 in, 6 out]
            n233 = call "Pin Positions DAO.vi"("LBCB Settings Actions"=w429, "LBCB Number"=w430) -> ("LBCB Pins Output"=w428:T14)  [unwired: 11 in, 2 out]
            n234 = call "Command Channel Names DAO.vi"("LBCB Number"=w430, "Actions"=w429) -> ("Names Out"=w444:T20)  [unwired: 3 in, 6 out]
            n235 = call "LVDT Channel Names DAO.vi"("LBCB Number"=w430, "Actions"=w429) -> ("Names Out"=w443:T20)  [unwired: 3 in, 6 out]
            n236 = call "Load Cell Channel Names DAO.vi"("LBCB Number"=w430, "Actions"=w429) -> ("Names Out"=w442:T20)  [unwired: 3 in, 6 out]
            n237 = call "Servo Error Channel Names DAO.vi"("LBCB Number"=w430, "Actions"=w429) -> ("Names Out"=w441:T20)  [unwired: 3 in, 6 out]
            n238 = local write "LBCB Pin Positions"(w428) -> ()
            n239 = local write "Command Channels"(w444) -> ()
            n240 = local write "LVDT Channels"(w443) -> ()
            n241 = local write "Load Cell Channels"(w442) -> ()
            n242 = local write "Servo Error  Channels"(w441) -> ()
            n243 = local write "Servo Error Offset"(w440) -> ()
            n244 = local write "External Sensor Specs"(w446) -> ()
          }
          frame "Exit" {
          }
        }
      }
      frame True {
      }
    }
  }
  n245 = Compound Arithmetic op=AND(w12, w11) -> (w10:bool)
  n246 = Not(x=w10) -> (.not. x?=w9:bool)
  n247 = flat-sequence {
    tunnel: w9 -> [w483]
    frame #0 {
      n248 = control-ref of="This VI"() -> (w482:refnum<vi>)
      n249 = invoke class="VI" method="FP.Close"(reference=w482) -> ()  [unwired: 2 in, 3 out]
      n250 = local write "Ok"(w483) -> ()
    }
  }
